vi "experiment.vi"(7 "Color":u32(colorbox)=14450432, 10 "new file":path=path "C:/Users/daniel.coons/Downloads/13mpmod.png", 11 "File Path":path=path "C:/Users/daniel.coons/Downloads/dark_mode_FILL0_wght300_GRAD200_opsz24.png") -> (0 "error out":errorcluster)   [LabVIEW 2021]
uses:
  System.Drawing
panel:
  out "ToString 2":string
  out "PropertyIdList 3":i32[](array[numeric])
  out "Value 2":u8[](array[numeric])
  out "Id":i32
  out "error out 2":errorcluster
  out "Value":u8[](array[numeric])
  out "PropertyIdList 2":i32[](array[numeric])
  out "PropertyIdList":i32[](array[numeric])
  out "Array 3":i32[](array[numeric]) format="%.0x"
  out "Array 2":u8[][](array[numeric])
  out "Array":i32[](array[numeric]) format="%.0x"
  out "Width":i32
  out "Height":i32
  out "ToString":string[](array[string])
  out "ToArgb":i32
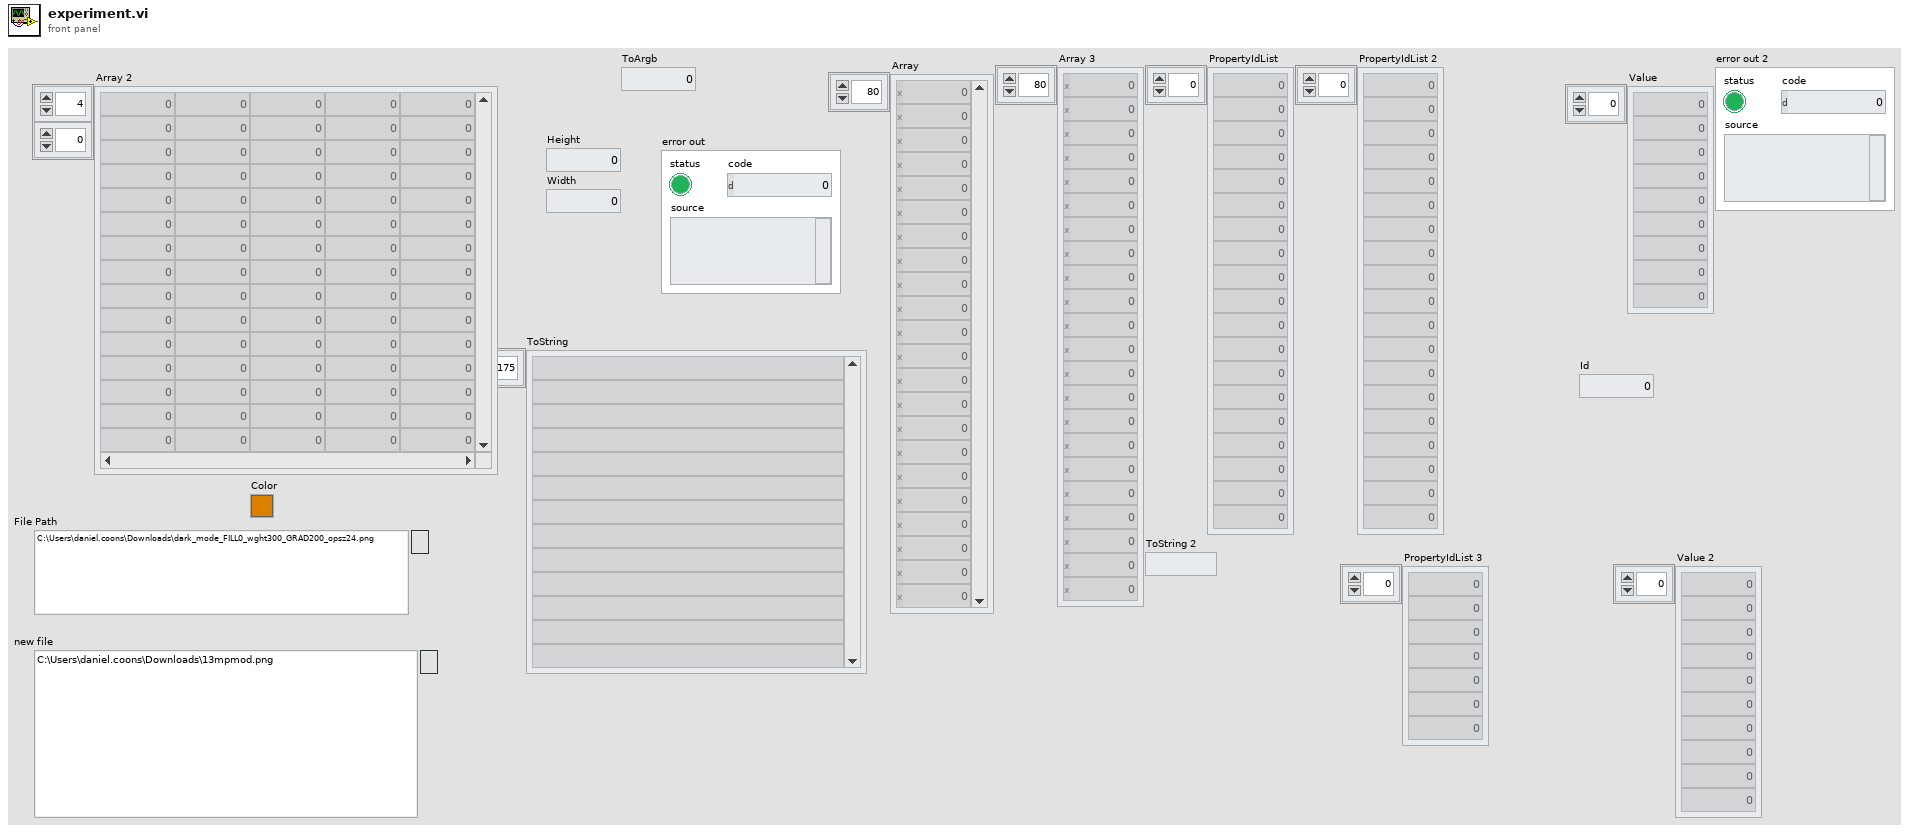
[diagram p1: front panel]
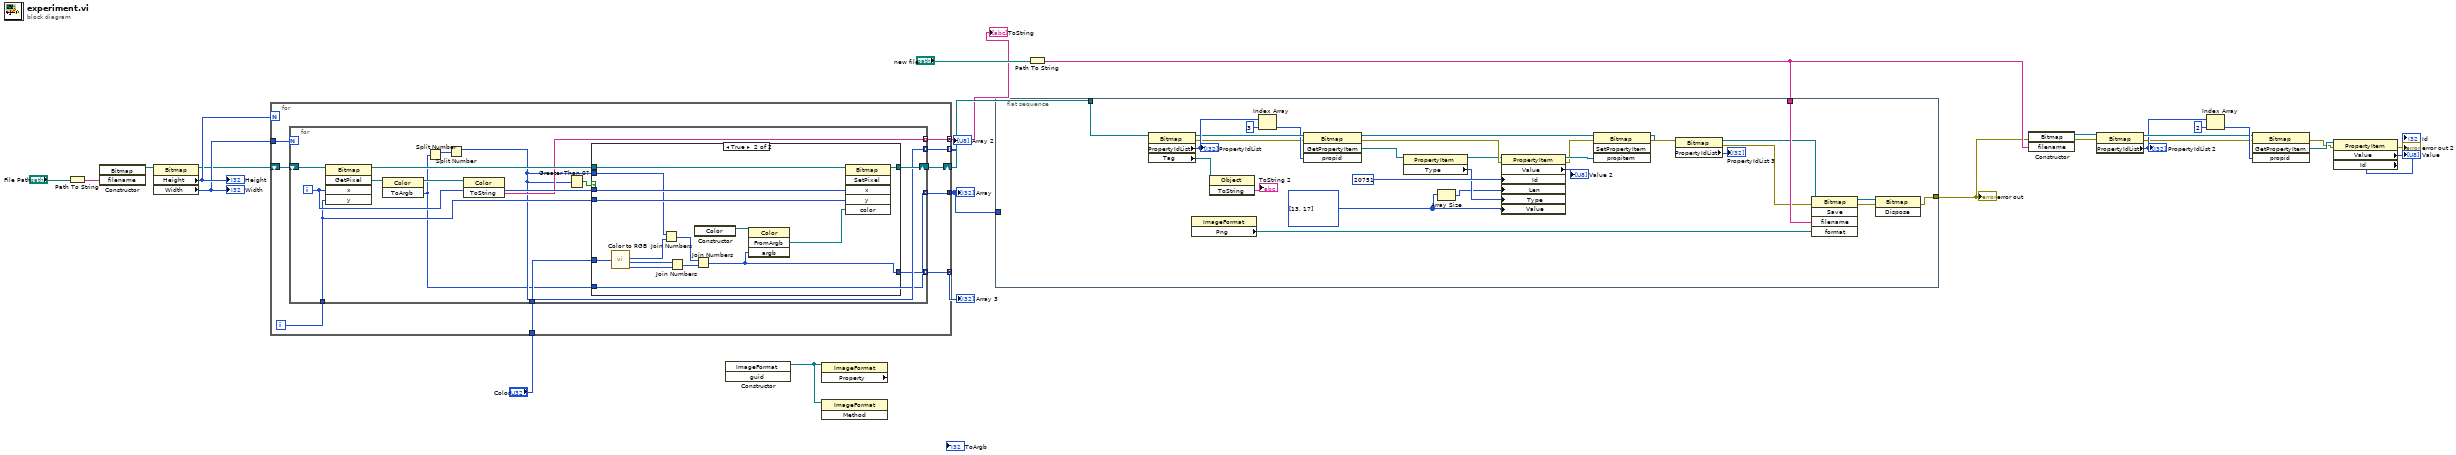
[diagram p0: block diagram]
diagram:
  n1 = Path To String(path="File Path") -> (string=w27:string)
  n2 = constructor class="Bitmap"("filename"=w27) -> (reference out=w26:refnum<k24>)  [unwired: 3 in, 3 out]
  n3 = property class="Bitmap"(reference=w26) -> (reference out=w23:refnum<k24>, "Height"=w25:i32, "Width"=w24:i32)  [unwired: 1 in, 1 out]
  "Height" <- w25
  "Width" <- w24
  n4 = for {
    N: w25 -> [_]
    tunnel: w24 -> [w37]
    tunnel: [w35] -> w22 mode=concatenating
    shift-right: [w33] -> w20
    shift-left: w23 -> [w34]
    tunnel: [w32] -> w19 mode=concatenating
    tunnel: [w31] -> w18 mode=indexing
    tunnel: "Color" -> [w30]
    tunnel: [w29] -> w16 mode=concatenating
    i -> [w36]
    n5 = for {
      N: w37 -> [_]
      tunnel: w36 -> [w47]
      tunnel: [w38] -> w35 mode=indexing
      shift-right: [w46] -> w33
      shift-left: w34 -> [w50]
      tunnel: [w44] -> w32 mode=indexing
      tunnel: [w41] -> w31 mode=indexing
      tunnel: w30 -> [w40]
      tunnel: [w39] -> w29 mode=indexing
      i -> [w48]
      n6 = invoke class="Bitmap" method="GetPixel"(reference=w50, "x"=w48, "y"=w47) -> (reference out=w49:refnum<k24>, "GetPixel"=w51:refnum<k24>)  [unwired: 2 in, 3 out]
      n7 = invoke class="Color" method="ToArgb"(reference=w51) -> (reference out=w45:refnum<k24>, "ToArgb"=w38:i32)  [unwired: 2 in, 1 out]
      n8 = Split Number(x=w38) -> (hi(x)=w43:u16)  [unwired: 1 out]
      n9 = Split Number(x=w43) -> (hi(x)=w41:u8)  [unwired: 1 out]
      n10 = invoke class="Color" method="ToString"(reference=w45) -> ("ToString"=w44:string)  [unwired: 2 in, 2 out]
      n11 = Greater Than 0?(x=w41) -> (x > 0?=w42:bool)
      n12 = case shown="True" w42 {
        tunnel: w49 -> [w53 w67]
        tunnel: w48 -> [_ w66]
        tunnel: w47 -> [_ w65]
        tunnel: [w53 w64] -> w46
        tunnel: w41 -> [_ w61]
        tunnel: w40 -> [_ w54]
        tunnel: [w52 w58] -> w39
        tunnel: w38 -> [w52 _]
        frame False {
        }
        frame True {
          n13 = call <vilib>:"Color to RGB.vi"("Color"=w54) -> ("R"=w57:u8, "G"=w56:u8, "B"=w55:u8)  [unwired: 1 out]
          n14 = Join Numbers(hi=w61, lo=w57) -> ((hi.lo)=w60:u16)
          n15 = Join Numbers(hi=w56, lo=w55) -> ((hi.lo)=w59:u16)
          n16 = constructor class="Color"() -> (reference out=w63:refnum<k24>)  [unwired: 3 in, 2 out]
          n17 = Join Numbers(hi=w60, lo=w59) -> ((hi.lo)=w58:u32)
          n18 = invoke class="Color" method="FromArgb"(reference=w63, "argb"=w58) -> ("FromArgb"=w62:refnum<k24>)  [unwired: 2 in, 3 out]
          n19 = invoke class="Bitmap" method="SetPixel"(reference=w67, "x"=w66, "y"=w65, "color"=w62) -> (reference out=w64:refnum<k24>)  [unwired: 2 in, 5 out]
        }
      }
    }
  }
  "Array" <- w22
  "ToString" <- w19
  "Array 2" <- w18
  "Array 3" <- w16
  n20 = constructor class="ImageFormat"() -> (reference out=w1:refnum<k24>)  [unwired: 4 in, 3 out]
  n21 = property class="ImageFormat" props=[](reference=w1) -> ()  [unwired: 1 in, 3 out]
  n22 = invoke class="ImageFormat" method=#-1(reference=w1) -> ()  [unwired: 2 in, 3 out]
  n23 = flat-sequence {
    tunnel: w20 -> [w93]
    tunnel: w22 -> [_]
    tunnel: w15 -> [w96]
    tunnel: [w76] -> w7
    frame #0 {
      w71 = u8[] [13, 17] ("Value")
      n24 = property class="Bitmap"(reference=w93) -> (reference out=w91:refnum<k24>, error out=w82:errorcluster, "PropertyIdList"=w92:i32[], "Tag"=w69:refnum<k24>)  [unwired: 1 in]
      "PropertyIdList" <- w92
      n25 = property class="ImageFormat"() -> ("Png"=w94:refnum<k24>)  [unwired: 2 in, 2 out]
      n26 = invoke class="Object" method="ToString"(reference=w69) -> ("ToString"=→"ToString 2":string)  [unwired: 2 in, 2 out]
      n27 = Index Array(array=w92, index=3) -> (element=w90:i32)
      n28 = invoke class="Bitmap" method="GetPropertyItem"(reference=w91, error in=w82, "propid"=w90) -> (reference out=w86:refnum<k24>, error out=w84:errorcluster, "GetPropertyItem"=w88:refnum<k24>)  [unwired: 1 in, 1 out]
      n29 = property class="PropertyItem"(reference=w88) -> (reference out=w73:refnum<k24>, "Type"=w72:i16)  [unwired: 1 in, 1 out]
      n30 = Array Size(array=w71) -> (size(s)=w70:i32)
      n31 = property class="PropertyItem"(reference=w73, error in=w84, "Id"=20751, "Len"=w70, "Type"=w72, "Value"=w71) -> (reference out=w87:refnum<k24>, error out=w83:errorcluster, "Value"=→"Value 2":u8[])
      n32 = invoke class="Bitmap" method="SetPropertyItem"(reference=w86, error in=w83, "propitem"=w87) -> (reference out=w79:refnum<k24>, error out=w85:errorcluster)  [unwired: 1 in, 2 out]
      n33 = property class="Bitmap"(reference=w79, error in=w85) -> (reference out=w78:refnum<k24>, error out=w80:errorcluster, "PropertyIdList"=→"PropertyIdList 3":i32[])
      n34 = invoke class="Bitmap" method="Save"(reference=w78, error in=w80, "filename"=w96, "format"=w94) -> (reference out=w75:refnum<k24>, error out=w95:errorcluster)  [unwired: 1 in, 3 out]
      n35 = invoke class="Bitmap" method="Dispose"(reference=w75, error in=w95) -> (error out=w76:errorcluster)  [unwired: 1 in, 2 out]
    }
  }
  n36 = Path To String(path="new file") -> (string=w15:string)
  n37 = constructor class="Bitmap"(error in=w7, "filename"=w15) -> (reference out=w10:refnum<k24>, error out=w5:errorcluster)  [unwired: 2 in, 2 out]
  n38 = property class="Bitmap"(reference=w10, error in=w5) -> (reference out=w12:refnum<k24>, error out=w4:errorcluster, "PropertyIdList"=w11:i32[])
  "PropertyIdList 2" <- w11
  n39 = Index Array(array=w11, index=2) -> (element=w13:i32)
  n40 = invoke class="Bitmap" method="GetPropertyItem"(reference=w12, error in=w4, "propid"=w13) -> (error out=w3:errorcluster, "GetPropertyItem"=w9:refnum<k24>)  [unwired: 1 in, 2 out]
  n41 = property class="PropertyItem"(reference=w9, error in=w3) -> (error out=→"error out 2":errorcluster, "Value"=→"Value":u8[], "Id"=→"Id":i32)  [unwired: 1 out]
  "error out" <- w7
